vi "RegisteredMessages.vi"() -> (3 "registered messages":string[](array[string]))   [LabVIEW 2017, in "IrDataEventCreator.lvlib"]
uses:
  <vilib>/addons/InsightCM/Devices/Shared/Ir/IrDataEventCreator/IrDataEventCreator.lvlib
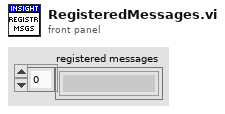
[diagram p1: front panel]
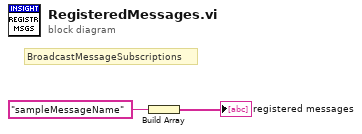
[diagram p0: block diagram]
diagram:
  # "BroadcastMessageSubscriptions"
  n1 = Build Array("sampleMessageName" ("String")) -> (→"registered messages":string[])
